vi "Configure OVP.vi"(8 "error in (no error)":errorcluster, 10 "SOVP":dbl format="%0.1f", 11 "VISA resource name":refnum<visa-resource-name>) -> (0 "error out":errorcluster, 3 "VISA resource name out":refnum<visa-resource-name>)   [LabVIEW 2021, in "BK Precision 169XB.lvlib"]
doc: "Configures over voltage protection (OVP) of the power supply. Specify the voltage limit and whether to enable or disable OVP."
uses:
  BK Precision 169XB.lvlib
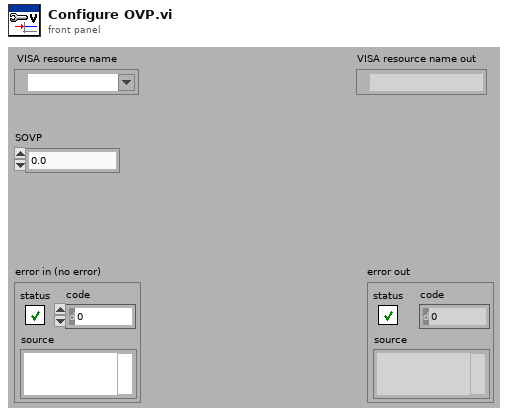
[diagram p1: front panel]
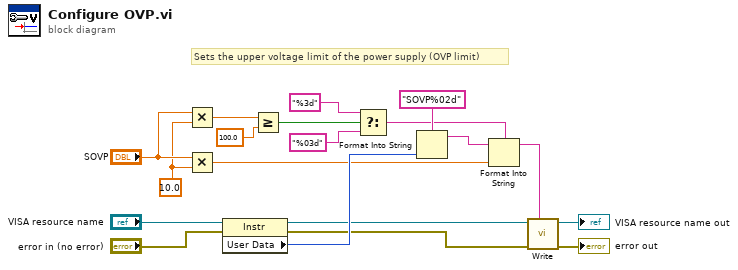
[diagram p0: block diagram]
diagram:
  w11 = 10.0 ("y")
  # "Sets the upper voltage limit of the power supply (OVP limit)"
  n1 = Multiply(x="SOVP", y=w11) -> (x*y=w19:dbl)
  n2 = Multiply(x="SOVP", y=w11) -> (x*y=w1:dbl)
  n3 = property class="Instr"(reference="VISA resource name", error in="error in (no error)") -> (reference out=w7:refnum<visa-resource-name>, error out=w6:errorcluster, "User Data"=w9:u32)
  n4 = Greater Or Equal?(x=w19, y=100.0) -> (x >= y?=w17:bool)
  n5 = Select(t="%3d" ("format string"), s=w17, f="%03d" ("format string")) -> (s? t:f=w4:string)
  n6 = Format Into String(format string="SOVP%02d" ("Enable/Disable Output"), w9) -> (resulting string=w3:string)  [unwired: 2 in, 1 out]
  n7 = Format Into String(format string=w4, initial string=w3, w1) -> (resulting string=w2:string)  [unwired: 1 in, 1 out]
  n8 = call "Write.vi"("Input String"=w2, "error in (no error)"=w6, "VISA resource name"=w7) -> ("error out"=→"error out":errorcluster, "VISA resource name out"=→"VISA resource name out":refnum<visa-resource-name>)  [unwired: 6 in, 1 out]
